vi "Constructor.vi"(8 "error in (no error)":errorcluster, 11 "AbstractModel in":refnum<class "AbstractModel.lvclass">) -> (0 "error out":errorcluster, 3 "AbstractModel out":refnum<class "AbstractModel.lvclass">)   [LabVIEW 2020, in "AbstractModel.lvclass"]
uses:
  AbstractModel.lvclass
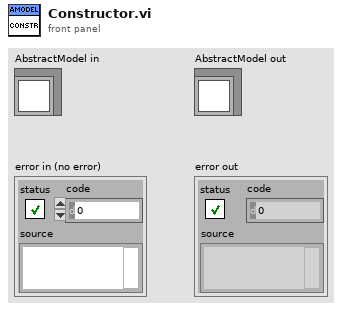
[diagram p1: front panel]
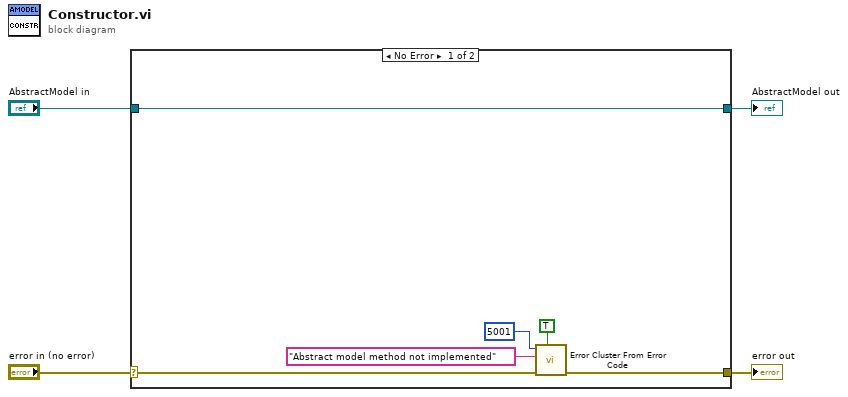
[diagram p0: block diagram]
diagram:
  n1 = case shown="No Error" "error in (no error)" {
    selector: "error in (no error)" -> [w6 w12]
    tunnel: [w5 w12] -> w3
    tunnel: [w10 w11] -> w1
    tunnel: "AbstractModel in" -> [w10 w11]
    frame No Error {
      n2 = call <vilib>:"Error Cluster From Error Code.vi"("show call chain? (False)"=TRUE, "error in (no error)"=w6, "error message (\"\")"="Abstract model method not implemented" ("error message (\"\")"), "error code (0)"=5001) -> ("error out"=w5:errorcluster)  [unwired: 5 in]
    }
    frame Error {
    }
  }
  "error out" <- w3
  "AbstractModel out" <- w1
